vi "SetParam.vi"(8 "error in (no error)":errorcluster caption="entrée d'erreur (pas d'erreur)", 10 "robust_scale":T1={"axis"=0, "with_centering"=TRUE, "with_scaling"=TRUE, "quantile_range"={"q_min"=25.0, "q_max"=75.0}, "copy"=TRUE}, 11 "robust_scale.lvclass":refnum<class "robust_scale.lvclass">) -> (0 "error out":errorcluster caption="sortie d'erreur", 3 "robust_scale.lvclass":refnum<class "robust_scale.lvclass">)   [LabVIEW 2020, in "robust_scale.lvclass"]
doc: "Set Parameters"
uses:
  robust_scale.lvclass
  robust_scale.lvclass/robust_scale.ctl
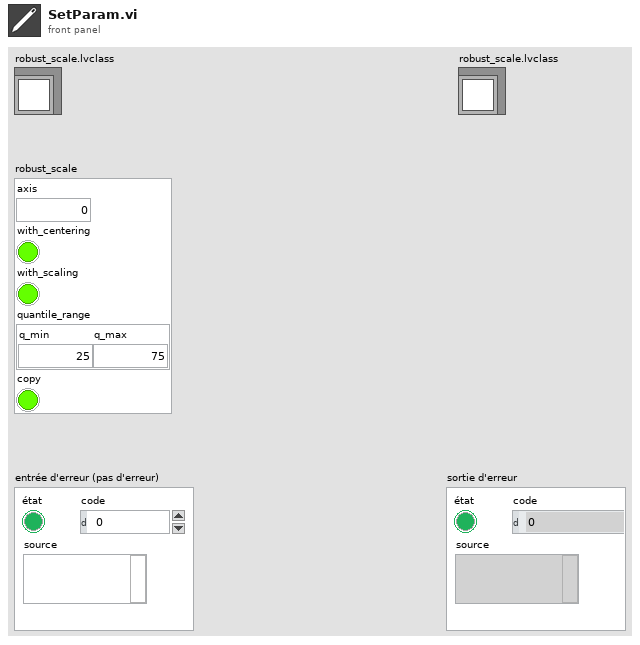
[diagram p1: front panel]
types:
  T1 = cluster{"axis":i32, "with_centering":bool, "with_scaling":bool, "quantile_range":cluster{"q_min":dbl, "q_max":dbl}, "copy":bool}
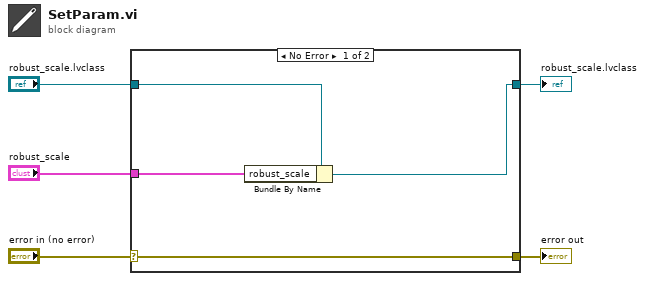
[diagram p0: block diagram]
diagram:
  n1 = case shown="No Error" "error in (no error)" {
    selector: "error in (no error)" -> [w9 w10]
    tunnel: [w9 w10] -> w4
    tunnel: [w7 w11] -> w2
    tunnel: "robust_scale.lvclass" -> [w8 w11]
    tunnel: "robust_scale" -> [w6 _]
    frame No Error {
      n2 = Bundle By Name(cluster=w8, "robust_scale"=w6) -> (w7:refnum<class "robust_scale.lvclass">)
    }
    frame Error {
    }
  }
  "error out" <- w4
  "robust_scale.lvclass" <- w2
